vi "WAVFiles.vi"(6 "Task":enum16{"Read", "Write", "wfm"}(ring), 8 "Data In":cluster{dbl, dbl, dbl[]}[](graph), 9 "Settings":T1={"Name of test"="", "Date"=timestamp(0 s since 1904-01-01), "Location"="", "Template"="", "Soundcard"="", "resolution"=32, "Sampling rate"=48000, "Ch1 Gain "=25.0, "Ch2 Gain"=10.0, "Sample time (s)"=0.3, "Pre-trigger (s)"=0.01, "Hammer Threshold"=10.0, "Positions"=12, "Taps/Position"=5, "Set Names"="", "Freq resolution"=10.0, "Hammer cutoff"=0.0, "Mic cutoff"=0.0, "Double bounce "=0.0, "Hammer Cal"=10.0, "dB Offset"=0.0, "Accel Cal"=10.0, "Vibrometer Cal"=0.0, "Mic Cal"=0.0, "Output"=2, "Voltage Cal"=1.0, "Vibrometer Port"="ASRL27::INSTR", "Range"=4, "High Pass"=2, "Bandwidth"=4, "X Range"=[], "Y Range"=[], "dB Spread"=0.0, "Trigger"=0, "Ch_1"=25, "Ch_2"=25, "flip?"=FALSE, "60Hz"=FALSE, "Time offset"=0.0, "Piezo Cal"=1.0, "Default Notes"=""} {"Ch_2" min=1 step=1; "Ch_1" min=1 max=100 step=1; "Trigger" items=["Hammer (force)", "Self-tap", "Spacebar"]; "Bandwidth" items=["1 kHz"=1, "5 kHz"=5, "10 kHz"=10, "25 kHz"=25, "50 kHz"=50, "100 kHz"=100]; "High Pass" items=["Off", "13 Hz", "104 Hz"]; "Range" items=["10 mm/s"=1, "20 mm/s"=2, "50 mm/s"=5, "100 mm/s"=10, "200 mm/s"=20, "500 mm/s"=50, "1 m/s"=100, "2 m/s"=200]; "Output" items=["Accelerometer", "Speed (from acceleration)", "Microphone", "Vibrometer", "Piezo"]; "Voltage Cal" format="%#_13g"; "Ch2 Gain" format="%#_13g"; "Ch1 Gain" format="%#_13g"; "Double bounce" min=0.0; "Mic cutoff" min=0.0 format="%#_4g"; "Hammer cutoff" min=0.0 format="%#_4g"; "Freq resolution" min=0.0; "Pre-trigger (s)" format="%#_13g"; "Date" format="%<%H:%M\n%d/%m/%y>T"; "resolution" items=["16 bit"=16, "24 bit"=24, "32 bit"=32]; "Sampling rate" items=["22050 samp/s"=22050, "44100 samp/s"=44100, "48000 samp/s"=48000]}, 10 "Wfm data":waveform(dbl)[](graph)=[{"t0"=timestamp(0 s since 1904-01-01), "dt"=2.2675736961451248e-05, "Y"=[0.0018600813345983624, 0.0013567095156759024, 0.000724937068298459, 0.0007585012936033309, 0.00165243458468467, 0.0020575118251144886, 0.0018339351518079638, 0.001325494609773159, 0.0009242118685506284, 0.0004103305109310895, 0.0014500700635835528, 0.0020430416334420443, 0.0010176138021051884, 0.0013936994364485145, 0.0021213560830801725, 0.001495259813964367, 0.0001298538554692641, 0.00048586272168904543, 0.0018768651643767953, 0.0012630799319595098]}, {"t0"=timestamp(0 s since 1904-01-01), "dt"=2.2675736961451248e-05, "Y"=[-0.0018600813345983624, -0.0013567095156759024, -0.000724937068298459, -0.0007585012936033309, -0.00165243458468467, -0.0020575118251144886, -0.0018339351518079638, -0.001325494609773159, -0.0009242118685506284, -0.0004103305109310895, -0.0014500700635835528, -0.0020430416334420443, -0.0010176138021051884, -0.0013936994364485145, -0.0021213560830801725, -0.001495259813964367, -0.0001298538554692641, -0.00048586272168904543, -0.0018768651643767953, -0.0012630799319595098]}], 11 "WAV File":path=path "/Users/crogers/Desktop/ObieDataSOtrage/32float.wav") -> (0 "error out":errorcluster, 1 "format":T2, 2 "Valid?":bool, 3 "Data":waveform(dbl)[](graph))   [LabVIEW 2022 SP3]
uses:
  PreferencesControl.ctl
panel:
  out "size(s)":i32
  out "File Size":u32
  # "Hz"
  # "dB"
  # "dB"
  # "sec"
  # "sec"
  # "mV/Pa"
  # "mV/m/s2"
  # "mV/mm/s"
  # "V/N"
  # "sec"
  # "sec"
  # "mV/N"
  # "a.u."
  # "a.u."
  # "sec"
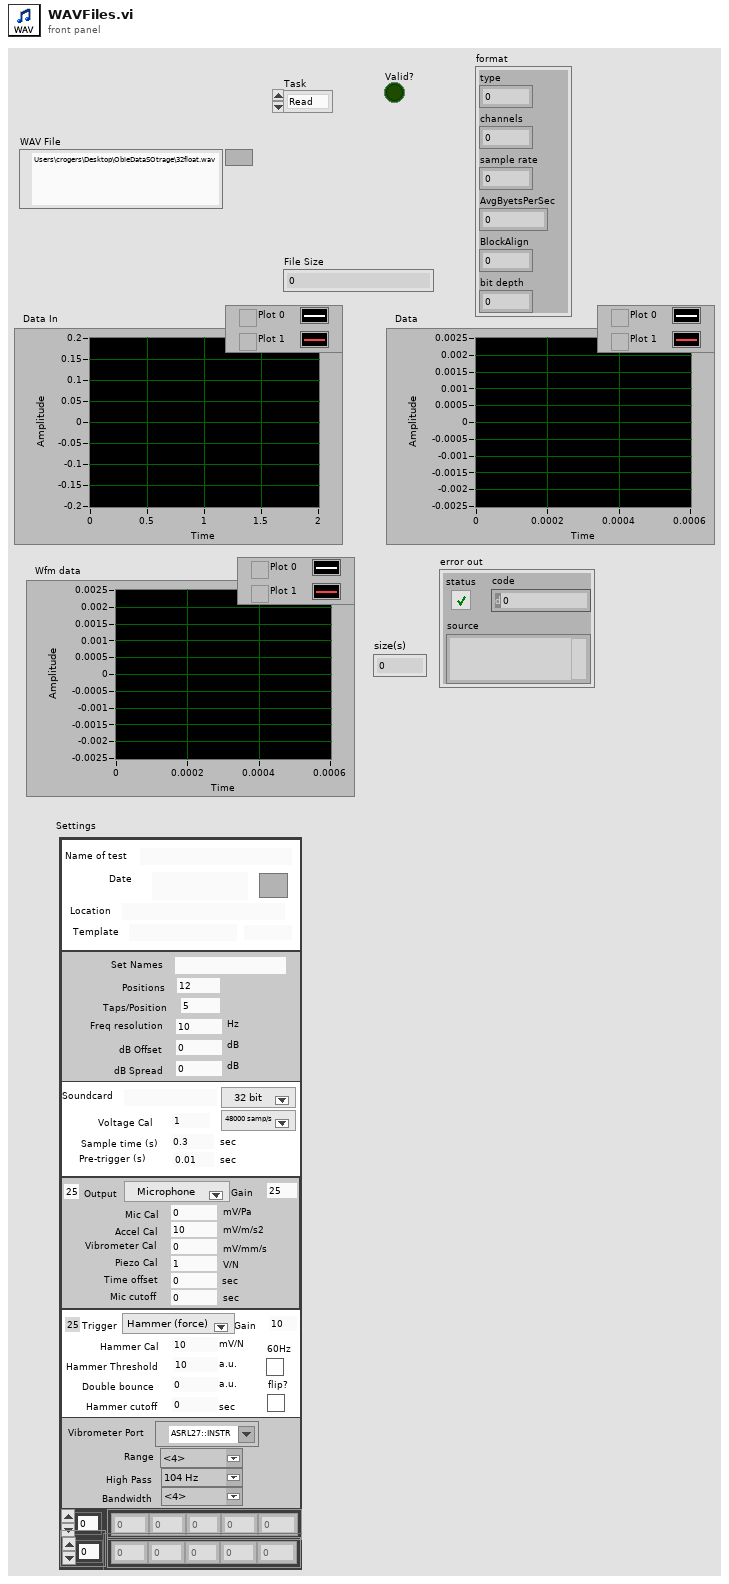
[diagram p1: front panel]
types:
  T1 = typedef "PreferencesControl.ctl" = cluster{"Name of test":string, "Date":timestamp, "Location":string, "Template":string, "Soundcard":string, "resolution":u16, "Sampling rate":u16, "Ch1 Gain ":dbl, "Ch2 Gain":dbl, "Sample time (s)":dbl, "Pre-trigger (s)":dbl, "Hammer Threshold":dbl, "Positions":i16, "Taps/Position":i16, "Set Names":string, "Freq resolution":dbl, "Hammer cutoff":dbl, "Mic cutoff":dbl, "Double bounce ":dbl, "Hammer Cal":dbl, "dB Offset":dbl, "Accel Cal":dbl, "Vibrometer Cal":dbl, "Mic Cal":dbl, "Output":u16, "Voltage Cal":dbl, "Vibrometer Port":refnum<visa-resource-name>, "Range":u16, "High Pass":u16, "Bandwidth":u16, "X Range":cluster{"Minimum":dbl, "Maximum":dbl, "Increment":dbl, "Minor Increment":dbl, "Start":dbl}[], "Y Range":cluster{"Minimum":dbl, "Maximum":dbl, "Increment":dbl, "Minor Increment":dbl, "Start":dbl}[], "dB Spread":dbl, "Trigger":u16, "Ch_1":u8, "Ch_2":u8, "flip?":bool, "60Hz":bool, "Time offset":dbl, "Piezo Cal":dbl, "Default Notes":string}
  T2 = cluster{"type":u16, "channels":u16, "sample rate":u32, "AvgByetsPerSec":u32, "BlockAlign":u16, "bit depth":u16}
  T3 = cluster{"Name":string, "Size":u32, "Contents":string}[]
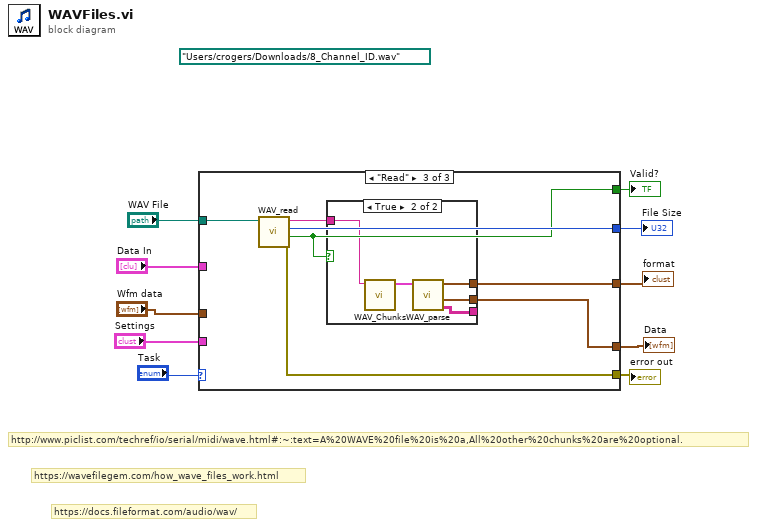
[diagram p0: block diagram]
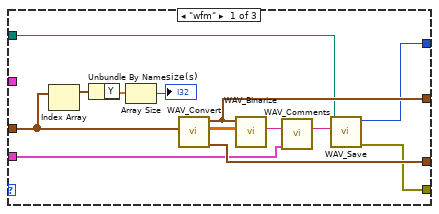
[diagram p2: hidden frame]
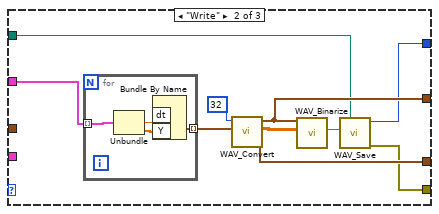
[diagram p3: hidden frame]
diagram:
  (unwired) path "/Users/crogers/Downloads/8_Channel_ID.wav" ("file (use dialog)")
  # "https://docs.fileformat.com/audio/wav/"
  # "https://wavefilegem.com/how_wave_files_work.html"
  # "http://www.piclist.com/techref/io/serial/midi/wave.html#:~:text=A%20WAVE%20file%20is%20a,All%20other%20chunks%20are%20optional."
  n1 = case shown="\"Read\"" "Task" {
    tunnel: [w18 w25 w44] -> w10
    tunnel: [w22 w31 w43] -> w9
    tunnel: [w20 w27 w40] -> w6
    tunnel: "WAV File" -> [w21 w30 w41]
    tunnel: [_ _ w38] -> w5
    tunnel: [w19 w26 w39] -> w4
    tunnel: "Wfm data" -> [w14 _ _]
    tunnel: "Data In" -> [_ w24 _]
    tunnel: "Settings" -> [w15 _ _]
    frame "wfm" {
      n2 = Index Array(array=w14) -> (element=w13:waveform(dbl))  [unwired: 1 in]
      n3 = Unbundle By Name(w13) -> ("Y"=w12:dbl[])
      n4 = Array Size(array=w12) -> (size(s)=→"size(s)":i32)
      n5 = call "WAV_Convert.vi"("data"=w14) -> (0:"Data"=w20:waveform(sgl)[], 2:"Data"=w23:sgl[][], "format"=w22:T2)  [unwired: 8 in]
      n6 = call "WAV_Binarize.vi"("Data in"=w23, "format"=w22) -> ("file string"=w17:string)  [unwired: 9 in]
      n7 = call "WAV_Comments.vi"("Settings"=w15, "string in"=w17) -> ("string out"=w16:string)  [unwired: 9 in]
      n8 = call "WAV_Save.vi"("file string"=w16, "file (use dialog)"=w21) -> ("error out"=w19:errorcluster, "File Size"=w18:i32)  [unwired: 8 in]
    }
    frame "Write" {
      n9 = for {
        tunnel: w24 -> [w37] mode=indexing
        tunnel: [w34] -> w29 mode=indexing
        n10 = Unbundle(w37) -> (w35:dbl, w36:dbl[])  [unwired: 1 out]
        n11 = Bundle By Name("dt"=w35, "Y"=w36) -> (w34:waveform(dbl))  [unwired: 1 in]
      }
      n12 = call "WAV_Convert.vi"("data"=w29, "bit depth"=u16 32) -> (0:"Data"=w27:waveform(sgl)[], 2:"Data"=w33:sgl[][], "format"=w31:T2)  [unwired: 7 in]
      n13 = call "WAV_Binarize.vi"("Data in"=w33, "format"=w31) -> ("file string"=w32:string)  [unwired: 9 in]
      n14 = call "WAV_Save.vi"("file string"=w32, "file (use dialog)"=w30) -> ("error out"=w26:errorcluster, "File Size"=w25:i32)  [unwired: 8 in]
    }
    frame "Read" {
      n15 = call "WAV_read.vi"("file (use dialog)"=w41) -> ("error out"=w39:errorcluster, "Valid?"=w38:bool, "File Size"=w44:u32, "string out"=w42:string)  [unwired: 7 in]
      n16 = case shown="True" w38 {
        tunnel: [_ w48] -> w43
        tunnel: w42 -> [_ w47]
        tunnel: [_ w46] -> w40
        tunnel: [_ w45] -> _
        frame False {
        }
        frame True {
          n17 = call "WAV_Chunks.vi"("contents"=w47) -> ("Chunks"=w49:T3)  [unwired: 10 in]
          n18 = call "WAV_parse.vi"("Chunks"=w49) -> ("Parameters"=w45:string[][], "Graph"=w46:waveform(dbl)[], "format"=w48:T2)  [unwired: 8 in]
        }
      }
    }
  }
  "File Size" <- w10
  "format" <- w9
  "Data" <- w6
  "Valid?" <- w5
  "error out" <- w4
